vi "PolyLegendre.vi"(1 "n":i32) -> (0 "Pn":dbl[](array[numeric]))   [LabVIEW 2010, in "NI_AALPro.lvlib"]
uses:
  NI_AALPro.lvlib
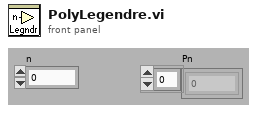
[diagram p1: front panel]
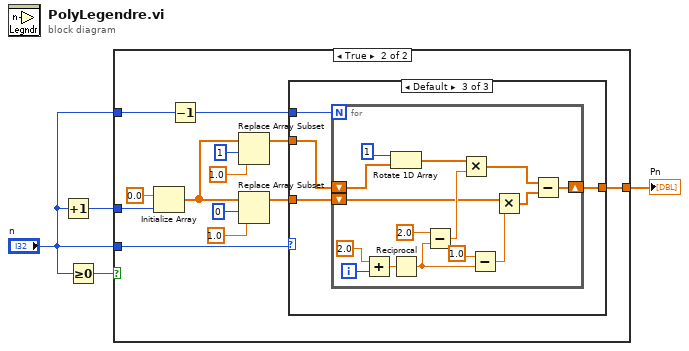
[diagram p0: block diagram]
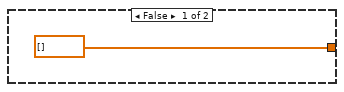
[diagram p2: hidden frame]
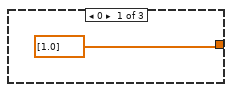
[diagram p3: hidden frame]
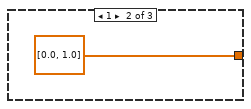
[diagram p4: hidden frame]
diagram:
  n1 = Increment(x="n") -> (x+1=w3:i32)
  n2 = Greater Or Equal To 0?(x="n") -> (x >= 0?=w4:bool)
  n3 = case shown="True" w4 {
    tunnel: "n" -> [_ w18]
    tunnel: w3 -> [_ w9]
    tunnel: "n" -> [_ w7]
    tunnel: [dbl[] [] ("Tn(x)") w8] -> w1
    frame False {
    }
    frame True {
      n4 = Initialize Array(0.0 ("element"), w9) -> (w15:dbl[])
      n5 = Decrement(x=w7) -> (x-1=w6:i32)
      n6 = Replace Array Subset(array=w15, new element=1.0 ("new element/subarray"), index=1) -> (w11:dbl[])
      n7 = Replace Array Subset(array=w15, new element=1.0 ("new element/subarray"), index=0) -> (w10:dbl[])
      n8 = case shown="Default" w18 {
        tunnel: w11 -> [_ _ w24]
        tunnel: w10 -> [_ _ w23]
        tunnel: w6 -> [_ _ w22]
        tunnel: [dbl[] [1.0] ("Tn(x)") dbl[] [0.0, 1.0] ("Tn(x)") w21] -> w8
        frame 0 {
        }
        frame 1 {
        }
        frame Default {
          n9 = for {
            N: w22 -> [_]
            shift-right: [w25] -> w21
            shift-left: w24 -> [w39]
            shift-left: w23 -> [w29]
            i -> [w37]
            n10 = Add(x=2.0, y=w37) -> (x+y=w35:dbl)
            n11 = Rotate 1D Array(1:w39, 2:1 ("n")) -> (0:w31:dbl[])
            n12 = Reciprocal(x=w35) -> (1/x=w33:dbl)
            n13 = Subtract(x=2.0, y=w33) -> (x-y=w30:dbl)
            n14 = Multiply(x=w31, y=w30) -> (x*y=w27:dbl[])
            n15 = Subtract(x=1.0, y=w33) -> (x-y=w28:dbl)
            n16 = Multiply(x=w29, y=w28) -> (x*y=w26:dbl[])
            n17 = Subtract(x=w27, y=w26) -> (x-y=w25:dbl[])
          }
        }
      }
    }
  }
  "Pn" <- w1
